vi "WhiteScreenTest_Startup.vi"() -> (0 "ErrorOut":errorcluster)   [LabVIEW 2018] (continued)
  w115 = "FPGA1" ("name (unnamed)")
  w161 = cluster{"QElmnt":T47, "Data":variant} {"QElmnt"=enum."Spvsr_InitQ", "Data"=variant} ("Cluster")
  # "Remove ATA_RF_Acquisition folder from path"
  # "Remove VI from path"
  # "Remove ATA_RF_Acquisition folder from path"
  # "Remove VI from path"
  # "Remove ATA_RF_Acquisition folder from path"
  # "Remove VI from path"
  # "Remove ATA_RF_Acquisition folder from path"
  # "Remove VI from path"
  # "Note that the Main Queue is made available to the HW Loop (and other loops) for things such as Error Handling as well as for allowing the HW Loop to drive information back up to the Main Loop for tasks such as refreshing panel controls  based on a change in HW State (\"Run\" to \"Pause\" or \"Waiting on Trigger\" to \"Triggered\")"
  # "The Hypervisor is optional and allows for data logging of user and other system events.  This can be expanded upon to be called from anywhere in the software depending on how detailed the event logging requirements of the application.\n\nThe data type defined for the queue allows for a string for event name, time, variant data type for longer descriptors or data and the stop condition but this can be expanded to allow for any number of variables to be written.\n\nWith each call to Add, an event is added to the Queue that needs to be read off and written.  The HypervisorWrite.vi is called in a parallel loop below to log these events as they are added to the queue."
  # "Copyright © 2017 Epimedia, Inc. All Rights Reserved.\n\nThe Epimedia Application Library is Copyright © 2009-2017 Epimedia, Inc. \nAll Rights Reserved. Used under license."
  # "Cluster data flow is predominantly top to bottom with data being passed using queues.  The Event Structure drives the Main (Consumer) Loop which acts as the Supervisor or dominant loop in this architecture.  In doing so, it handles the functionality of the other loops in your program.  The Consumer Loop processes the 'event' and then if necessary, sends the Master Cluster or a sub-cluster by means of a queue down to the Hardware Loop.  The Hardware loop checks the queued event's data for new information and if there is none, uses the previous iteration's cluster from the Shift Register.  Depending on the mode/event of the Hardware loop, the Hardware Loop may need to update the Master Cluster and does so by pushing the Refresh Panel Queue event which passes the cluster up to the Consumer loop for processing and panel update.  Note that there is a Functional Global inside of the UpdateMasterCluster.vi that is used to maintain a copy of the Master Cluster in memory that can be accessed from anywhere in the software (subVIs included).  This is not always and is often quite unnecessary, but is shown to illustrate a way of passing data between loops without using a Queue.  This use of a FG is quite effective, but must be used with care in that you need to be cautious with where and how often you update the FG; too many writers can cause unpredictable and very challenging code to debug.  The Functional Global exists to allow for any point anywhere in the program and in any loop to grab a copy of your cluster.  This architecture is intended to be a solid starting point for most applications, but you will need to configure and tailor the framework for your specific application and the use of some of the concepts shown herein cannot and should not always be used precisely as shown or at all.\n\nGeneral Rules:\n\n- Don't touch your Hardware anywhere except the HW loop.\n- Try to dedicate loops to very specific tasks to compartmentalize your code as much as possible as this helps with readability and scalability.\n- Any and all periodic updates (logging to disk, graph updates to name two) should occur only in the GUI loop.  Periodic updates of front panel indicators in any other loop will cause unnecessary loop cycles.\n- State changes for the program (ie. Idle, Run, Stop, Error) are handled in the Main Loop only and the panel is updated accordingly. \n- Use the Refresh Panel case in the Main Loop to handle all state changes and Panel GUI configuration tasks (enable/disable controls, visible, colors, alarming, status indicators, etc.).\n- Most loops only run when called by event/queue at the prescribed rate of the software.  Depending on your application, timed or free-wheeling loops could be implemented here if desired, but free-wheeling loops can be inefficient if not carefully implemented.\n- There are a couple of cases such as InitSW that are currently only called upon initialization and never again as shown below and one could argue that they could be outside of the architecture, but if they are called once, they may need to be again, so it is helpful to include them in the overall architecture for potential future use.  An example of this would be InitHW as in the event of a HW failure resulting from poor configuration choices, it would be helpful to be able to call the InitHW case again to reinitialize the HW with new settings."
  n1 = Current VI's Path() -> (path=w75:path)
  n2 = Current VI's Path() -> (path=w81:path)
  n3 = Strip Path(path=w75) -> (stripped path=w74:path)  [unwired: 1 out]
  n4 = Strip Path(path=w81) -> (stripped path=w80:path)  [unwired: 1 out]
  n5 = Strip Path(path=w74) -> (stripped path=w73:path)  [unwired: 1 out]
  n6 = Current VI's Path() -> (path=w91:path)
  n7 = Current VI's Path() -> (path=w83:path)
  n8 = Strip Path(path=w80) -> (stripped path=w79:path)  [unwired: 1 out]
  n9 = Strip Path(path=w91) -> (stripped path=w90:path)  [unwired: 1 out]
  n10 = Strip Path(path=w83) -> (stripped path=w84:path)  [unwired: 1 out]
  n11 = flat-sequence {
    tunnel: [w166] -> w111
    tunnel: errorcluster {"status"=FALSE, "code"=0, "source"=""} ("ErrorIn") -> [w165]
    frame #0 {
      n12 = shared-variable ".\\Connex_Variables.lvlib\\10Hz_File_Refs"(T48 {"72Co_dset"=0, "84Co_dset"=0, "FileRef"=0} ("10Hz_File_Refs"), error in=w165) -> (error out=w166:errorcluster)
      n13 = local write "Exit"(FALSE ("Exit")) -> ()
    }
  }
  n14 = Strip Path(path=w90) -> (stripped path=w89:path)  [unwired: 1 out]
  n15 = Strip Path(path=w84) -> (stripped path=w85:path)  [unwired: 1 out]
  n16 = control-ref of="Power History 72 Co"() -> (w93:refnum<vi>)
  n17 = control-ref of="Power History 72 X"() -> (w94:refnum<vi>)
  n18 = control-ref of="Power History 84 Co"() -> (w95:refnum<vi>)
  n19 = control-ref of="Power History 84 X"() -> (w96:refnum<vi>)
  n20 = Build Path(base path=w79, name or relative path="NASA\\wtle_young_weather_stn\\WeatherStationMain_20180517.vi") -> (appended path=w77:path)
  n21 = Build Path(base path=w73, name or relative path="NASA\\statmon_2015\\ADAM_health_subpanel_20190329.vi") -> (appended path=w71:path)
  n22 = Obtain Queue(max queue size (-1, unlimited)=100, name (unnamed)="Supervisor", element data type=w161, error in (no error)=w111) -> (queue out=w162:refnum<queue>, error out=w163:errorcluster)  [unwired: 1 in, 1 out]
  n23 = Build Array(w93, w94, w95, w96) -> (w92:refnum<vi>[])
  n24 = Build Path(base path=w89, name or relative path="Disdrometer\\disdrometer_2020_09_09.vi") -> (appended path=w87:path)
  n25 = Build Path(base path=w85, name or relative path="NASA\\te_2015\\te_20200903.vi") -> (appended path=w82:path)
  n26 = Enqueue Element(queue=w162, element=w161, error in (no error)=w163) -> (queue out=w144:refnum<queue>, error out=w57:errorcluster)  [unwired: 2 out]
  n27 = Open VI Reference(vi path=w71, error in (no error)=w57) -> (vi reference=w63:refnum<vi>, error out=w30:errorcluster)  [unwired: 4 in]
  n28 = Open VI Reference(vi path=w87, error in (no error)=w57) -> (vi reference=w62:refnum<vi>, error out=w45:errorcluster)  [unwired: 4 in]
  n29 = Open VI Reference(vi path=w82, error in (no error)=w57) -> (vi reference=w61:refnum<vi>, error out=w28:errorcluster)  [unwired: 4 in]
  n30 = Open VI Reference(vi path=w77, error in (no error)=w57) -> (vi reference=w4:refnum<vi>, error out=w16:errorcluster)  [unwired: 4 in]
  n31 = invoke on="DisdroPanel" class="SubPnl" method="Insert VI"(error in=w45, "VI Ref"=w62) -> (error out=w42:errorcluster)  [unwired: 2 in, 3 out]
  n32 = invoke on="TE_panel" class="SubPnl" method="Insert VI"(error in=w28, "VI Ref"=w61) -> (error out=w18:errorcluster)  [unwired: 2 in, 3 out]
  n33 = invoke on="Sub Panel - Weather" class="SubPnl" method="Insert VI"(error in=w16, "VI Ref"=w4) -> (error out=w6:errorcluster)  [unwired: 2 in, 3 out]
  n34 = Obtain Queue(max queue size (-1, unlimited)=100, name (unnamed)="Data", element data type=w118, error in (no error)=w57) -> (queue out=w122:refnum<queue>, error out=w120:errorcluster)  [unwired: 1 in, 1 out]
  n35 = Obtain Queue(max queue size (-1, unlimited)=110, name (unnamed)="FP", element data type=w97, error in (no error)=w57) -> (queue out=w100:refnum<queue>, error out=w99:errorcluster)  [unwired: 1 in, 1 out]
  n36 = invoke on="ADAM Health" class="SubPnl" method="Insert VI"(error in=w30, "VI Ref"=w63) -> (error out=w29:errorcluster)  [unwired: 2 in, 3 out]
  n37 = Obtain Queue(max queue size (-1, unlimited)=100, name (unnamed)=w115, element data type=cluster{"HWMd":T27, "Data":variant} {"HWMd"=enum."HW_Init", "Data"=variant}, error in (no error)=w57) -> (queue out=w150:refnum<queue>, error out=w149:errorcluster)  [unwired: 1 in, 1 out]
  n38 = Obtain Queue(max queue size (-1, unlimited)=100, name (unnamed)=w114, element data type=cluster{"HWMd":T27, "Data":variant} {"HWMd"=enum."HW_Init", "Data"=variant}, error in (no error)=w57) -> (queue out=w53:refnum<queue>, error out=w131:errorcluster)  [unwired: 1 in, 1 out]
  n39 = Enqueue Element(queue=w122, element=w118, error in (no error)=w120) -> (queue out=w121:refnum<queue>, error out=w119:errorcluster)  [unwired: 1 in, 1 out]
  n40 = Obtain Queue(max queue size (-1, unlimited)=100, name (unnamed)="10Hz", element data type=cluster{"Enum":T23, "Var":variant} {"Enum"=enum."10Hz_Init", "Var"=variant}) -> (queue out=w2:refnum<queue>, error out=w3:errorcluster)  [unwired: 2 in, 1 out]
  n41 = Obtain Queue(max queue size (-1, unlimited)=1000, name (unnamed)="Tones", element data type=cluster{"Enum":T46, "Data":variant} {"Enum"=enum."Data_Init", "Data"=variant}, error in (no error)=w57) -> (queue out=w145:refnum<queue>, error out=w156:errorcluster)  [unwired: 1 in, 1 out]
  n42 = Obtain Queue(max queue size (-1, unlimited)=100, name (unnamed)="Digi", element data type=w124, error in (no error)=w57) -> (queue out=w128:refnum<queue>, error out=w126:errorcluster)  [unwired: 1 in, 1 out]
  n43 = Obtain Queue(max queue size (-1, unlimited)=100, name (unnamed)="Log", element data type=w65, error in (no error)=w57) -> (queue out=w67:refnum<queue>, error out=w69:errorcluster)  [unwired: 1 in, 1 out]
  n44 = Enqueue Element(queue=w100, element=w97, error in (no error)=w99) -> (queue out=w70:refnum<queue>, error out=w98:errorcluster)  [unwired: 1 in, 1 out]
  n45 = Enqueue Element(queue=w67, element=w65, error in (no error)=w69) -> (queue out=w66:refnum<queue>, error out=w68:errorcluster)  [unwired: 1 in, 1 out]
  n46 = invoke class="VI" method="Run VI"(reference=w4, error in=w6, "Wait until done"=FALSE ("Wait Until Done"), "Auto Dispose Ref"=FALSE ("Auto Dispose Reference")) -> (error out=w5:errorcluster)  [unwired: 1 in, 4 out]
  n47 = invoke class="VI" method="Run VI"(reference=w63, error in=w29, "Wait until done"=FALSE ("Wait Until Done"), "Auto Dispose Ref"=FALSE ("Auto Dispose Reference")) -> (error out=w31:errorcluster)  [unwired: 1 in, 4 out]
  n48 = invoke class="VI" method="Run VI"(reference=w62, error in=w42, "Wait until done"=FALSE ("Wait Until Done"), "Auto Dispose Ref"=FALSE ("Auto Dispose Reference")) -> (error out=w41:errorcluster)  [unwired: 1 in, 4 out]
  n49 = invoke class="VI" method="Run VI"(reference=w61, error in=w18, "Wait until done"=FALSE ("Wait Until Done"), "Auto Dispose Ref"=FALSE ("Auto Dispose Reference")) -> (error out=w17:errorcluster)  [unwired: 1 in, 4 out]
  n50 = Enqueue Element(queue=w128, element=w124, error in (no error)=w126) -> (queue out=w127:refnum<queue>, error out=w125:errorcluster)  [unwired: 1 in, 1 out]
  n51 = call "NoiseLoop.vi"("error in (no error)"=w119, "Queue in"=w121) -> ("error out"=w143:errorcluster)  [unwired: 9 in]
  n52 = disable-structure shown="Enabled" {
    disable-tunnel: [w173 w174] -> w117
    disable-tunnel: [w170 w174] -> w110
    disable-tunnel: w57 -> [w169 w174]
    frame Enabled {
      n53 = call "AI_Loop.vi"("error in"=w169, "AI_Type"=AI_Type_Enum."AI") -> ("error out"=w173:errorcluster)  [unwired: 9 in]
      n54 = call "AI_Loop.vi"("error in"=w169, "AI_Type"=AI_Type_Enum."TC") -> ("error out"=w170:errorcluster)  [unwired: 9 in]
    }
    frame Disabled {
    }
  }
  n55 = disable-structure shown="Enabled" {
    disable-tunnel: [w176 w177] -> w108
    disable-tunnel: w57 -> [w175 w177]
    frame Enabled {
      n56 = call "AO_Loop.vi"("error"=w175) -> ("error out"=w176:errorcluster)  [unwired: 10 in]
    }
    frame Disabled {
    }
  }
  n57 = call "LogLoop_HDF5_20190307.vi"("error in"=w68, "Queue in"=w66) -> ("error out"=w107:errorcluster)  [unwired: 9 in]
  n58 = call "DigitalOutput.vi"("error in (no error)"=w125, "Queue in"=w127) -> ("error out"=w116:errorcluster)  [unwired: 9 in]
  n59 = call "10HzLogLoop_HDF5_20210610.vi"("error in"=w3, "queue in"=w2) -> ("error out"=w54:errorcluster)  [unwired: 9 in]
  n60 = while {
    tunnel: w57 -> [w180]
    tunnel: [w178] -> w104
    stop <- w183 stop-if-true
    n61 = call "Elapsed Time"("Time Target (s)"="MemoryPlotRate") -> ("Time has Elapsed"=w182:bool)  [unwired: 11 in, 7 out]
    n62 = Wait Until Next ms Multiple(millisecond multiple=u32 50) -> ()  [unwired: 1 out]
    n63 = case shown="True" w182 {
      tunnel: w180 -> [w184 w187]
      tunnel: [w184 w185] -> w178
      frame False {
      }
      frame True {
        n64 = constructor class="Process"(error in=w187) -> (reference out=w197:refnum<k24>, error out=w188:errorcluster)  [unwired: 2 in, 1 out]
        n65 = invoke class="Process" method="GetCurrentProcess"(reference=w197, error in=w188) -> (reference out=w195:refnum<k24>, error out=w196:errorcluster, "GetCurrentProcess"=w189:refnum<k24>)  [unwired: 1 in]
        n66 = property class="Process"(reference=w189, error in=w196) -> (reference out=w193:refnum<k24>, error out=w192:errorcluster, "WorkingSet"=w190:i32)
        n67 = Divide(x=w190, y=i64 1024) -> (x/y=→"Memory Used By LV (KB)" →"Memory Used":dbl)
        n68 = Close Reference(reference=w193, error in (no error)=w192) -> (error out=w194:errorcluster)
        n69 = Close Reference(reference=w195, error in (no error)=w194) -> (error out=w185:errorcluster)
      }
    }
    n70 = local read "Exit"() -> (w183:bool)
  }
  n71 = call "TonesLoop_20190705.vi"("WeightOfNewFrequency"=1.0, "error in"=w156, "Queue in"=w145) -> ("error out"=w146:errorcluster)  [unwired: 8 in]
  n72 = while {
    tunnel: w144 -> [w201]
    shift-right: [w200] -> w155
    shift-left: w57 -> [w202]
    stop <- w199 stop-if-true
    n73 = event shown="[14] \"Exit\": Value Change;  Panel Close" {
      selector: _ -> [_ _ _ _ _ _ _ _ _ _ _ _ _ _ _]
      dyn-events: _ -> [_ _ _ _ _ _ _ _ _ _ _ _ _ _ _]
      timeout: 100 -> [_ _ _ _ _ _ _ _ _ _ _ _ _ _ _]
      tunnel: w202 -> [w207 w211 w220 w228 w234 w236 w240 w248 w256 w264 w267 w272 w276 w280 w284]
      tunnel: w201 -> [_ w218 w221 w223 w229 w237 w241 w249 w257 w265 w269 w273 w277 w281 w286]
      tunnel: [w207 w210 w222 w224 w230 w235 w239 w247 w255 w263 w268 w271 w275 w282 w285] -> w200
      tunnel: [_ w209 _ _ _ _ _ _ _ _ _ _ _ _ TRUE] -> w199
      event Timeout {
        # "13:24:24.3\n05/31/2018"
        # "Timeout Case is used to update 'heartbeat' clock on the front panel to provide an indication that the software is still running"
        n74 = event-data() -> ()  [unwired: 2 out]
        n75 = Get Date/Time In Seconds() -> (seconds since 1Jan1904=w206:timestamp)
        n76 = Format Date/Time String(time format string (%c)="%H:%M:%S%1u\n%m/%d/%Y", seconds (now)=w206, UTC format=TRUE) -> (date/time string=→"UTC date/time":string)
      }
      event Menu Selection (User) {
        # "This handles a menu selection while the program is running."
        n77 = event-data() -> ("ItemTag"=w212:string)  [unwired: 1 out]
        n78 = Scan From String(input string=w212, error in=w211, default 1=MainQueueElements."Spvsr_InitQ" ("QElmnt")) -> (error out=w208:errorcluster, output 1=w216:T47)  [unwired: 2 in, 2 out]
        n79 = Bundle(cluster=cluster{"QElmnt":T47, "Data":variant} {"QElmnt"=enum."Spvsr_InitQ", "Data"=variant} ("Cluster"), "QElmnt"=w216) -> (w215:cluster{"QElmnt":T47, "Data":variant})  [unwired: 1 in]
        n80 = Enqueue Element(queue=w218, element=w215, error in (no error)=w208) -> (error out=w210:errorcluster)  [unwired: 3 out]
        n81 = Equal?(x=MainQueueElements."Spvsr_Exit" ("QElmnt"), y=w216) -> (x = y?=w209:bool)
      }
      event Value Change {
        n82 = event-data() -> ()  [unwired: 2 out]
        n83 = Enqueue Element(queue=w221, element=cluster{"QElmnt":T51, "Data":variant} {"QElmnt"=enum."Spvsr_DigiOut", "Data"=variant} ("Cluster"), error in (no error)=w220) -> (error out=w222:errorcluster)  [unwired: 3 out]
      }
      event "Config": Value Change {
        n84 = event-data() -> ()  [unwired: 2 out]
        n85 = Enqueue Element(queue=w223, element=cluster{"QElmnt":T47, "Data":variant} {"QElmnt"=enum."Spvsr_Config", "Data"=variant} ("Cluster"), error in (no error)=w228) -> (error out=w225:errorcluster)  [unwired: 3 out]
        n86 = Enqueue Element(queue=w223, element=cluster{"QElmnt":T47, "Data":variant} {"QElmnt"=enum."Spvsr_FPConfig", "Data"=variant} ("Cluster"), error in (no error)=w225) -> (error out=w224:errorcluster)  [unwired: 3 out]
      }
      event "AutoOffset": Value Change {
        n87 = event-data() -> ()  [unwired: 2 out]
        n88 = Enqueue Element(queue=w229, element=cluster{"QElmnt":T47, "Data":variant} {"QElmnt"=enum."Spvsr_DigitzOffs", "Data"=variant} ("Cluster"), error in (no error)=w234) -> (error out=w231:errorcluster)  [unwired: 3 out]
        n89 = Enqueue Element(queue=w229, element=cluster{"QElmnt":T47, "Data":variant} {"QElmnt"=enum."Spvsr_FPConfig", "Data"=variant} ("Cluster"), error in (no error)=w231) -> (error out=w230:errorcluster)  [unwired: 3 out]
      }
      event "FreqsToRemove", "AvgAvg", "SNR_Thresh", "Width [bins]", "FreqsToRemove 2", "Width 2 [bins]", "SimulateFPGA": Value Change {
        n90 = event-data() -> ()  [unwired: 2 out]
        n91 = Enqueue Element(queue=w237, element=cluster{"QElmnt":T47, "Data":variant} {"QElmnt"=enum."Spvsr_FPConfig", "Data"=variant} ("Cluster"), error in (no error)=w236) -> (error out=w235:errorcluster)  [unwired: 3 out]
      }
      event "MaxTrackRate": Value Change {
        n92 = event-data() -> ()  [unwired: 6 out]
        n93 = for {
          tunnel: cluster{"QElmnt":T47, "Data":variant}[] [{"QElmnt"=enum."Spvsr_FPConfig", "Data"=variant}, {"QElmnt"=enum."Spvsr_TrackRate", "Data"=variant}] ("Cluster") -> [w245] mode=indexing
          tunnel: w241 -> [w244]
          shift-right: [w243] -> w239
          shift-left: w240 -> [w246]
          n94 = Enqueue Element(queue=w244, element=w245, error in (no error)=w246) -> (error out=w243:errorcluster)  [unwired: 3 out]
        }
      }
      event "AutoCenter": Value Change {
        n95 = event-data() -> ()  [unwired: 6 out]
        n96 = for {
          tunnel: cluster{"QElmnt":T47, "Data":variant}[] [{"QElmnt"=enum."Spvsr_FPConfig", "Data"=variant}, {"QElmnt"=enum."Spvsr_AutoCenter", "Data"=variant}] ("Cluster") -> [w253] mode=indexing
          tunnel: w249 -> [w252]
          shift-right: [w251] -> w247
          shift-left: w248 -> [w254]
          n97 = Enqueue Element(queue=w252, element=w253, error in (no error)=w254) -> (error out=w251:errorcluster)  [unwired: 3 out]
        }
      }
      event "base path", "NAS path", "ThreshFile", "Location": Value Change {
        n98 = event-data() -> ()  [unwired: 6 out]
        n99 = for {
          tunnel: cluster{"QElmnt":T47, "Data":variant}[] [{"QElmnt"=enum."Spvsr_FPConfig", "Data"=variant}, {"QElmnt"=enum."Spvsr_RestartWarn", "Data"=variant}] ("Cluster") -> [w261] mode=indexing
          tunnel: w257 -> [w260]
          shift-right: [w259] -> w255
          shift-left: w256 -> [w262]
          n100 = Enqueue Element(queue=w260, element=w261, error in (no error)=w262) -> (error out=w259:errorcluster)  [unwired: 3 out]
        }
      }
      event "Beacon", "Beacon 3": Cursor Move {
        n101 = event-data() -> ()  [unwired: 2 out]
        n102 = Enqueue Element(queue=w265, element=cluster{"QElmnt":T47, "Data":variant} {"QElmnt"=enum."Spvsr_Cursors", "Data"=variant} ("Cluster"), error in (no error)=w264) -> (error out=w263:errorcluster)  [unwired: 3 out]
      }
      event "noise_ctrl", "72GHz_ctrl", "84GHz_ctrl": Value Change {
        n103 = event-data() -> ()  [unwired: 6 out]
        n104 = Enqueue Element(queue=w269, element=cluster{"QElmnt":T47, "Data":variant} {"QElmnt"=enum."FP_AO_ctrl", "Data"=variant} ("Cluster"), error in (no error)=w267) -> (error out=w268:errorcluster)  [unwired: 3 out]
      }
      event "Zoom On Peak", "AutoScale Y Noise", "AutoScale Y Tones": Value Change {
        n105 = event-data() -> ()  [unwired: 2 out]
        n106 = Enqueue Element(queue=w273, element=cluster{"QElmnt":T47, "Data":variant} {"QElmnt"=enum."Spvsr_FPConfig", "Data"=variant} ("Cluster"), error in (no error)=w272) -> (error out=w271:errorcluster)  [unwired: 3 out]
      }
      event Value Change {
        n107 = event-data() -> ()  [unwired: 6 out]
        n108 = Enqueue Element(queue=w277, element=cluster{"QElmnt":T47, "Data":variant} {"QElmnt"=enum."Spvsr_AlarmCfg", "Data"=variant} ("Cluster"), error in (no error)=w276) -> (error out=w275:errorcluster)  [unwired: 3 out]
      }
      event "Stop": Value Change {
        n109 = event-data() -> ()  [unwired: 2 out]
        n110 = Enqueue Element(queue=w281, element=cluster{"QElmnt":T47, "Data":variant} {"QElmnt"=enum."Spvsr_Stop", "Data"=variant} ("Cluster"), error in (no error)=w280) -> (error out=w282:errorcluster)  [unwired: 3 out]
      }
      event "Exit": Value Change; Panel Close {
        n111 = event-data() -> ()  [unwired: 2 out]
        n112 = Enqueue Element(queue=w286, element=cluster{"QElmnt":T47, "Data":variant} {"QElmnt"=enum."Spvsr_Exit", "Data"=variant} ("Cluster"), error in (no error)=w284) -> (error out=w285:errorcluster)  [unwired: 3 out]
      }
    }
  }
  n113 = while {
    shift-right: [w301] -> w154
    shift-left: w57 -> [w300]
    tunnel: w144 -> [w291]
    shift-right: [w302] -> _
    shift-left: T32 {"Admin"={"Lvl"=enum."Admin", "Pwd"=""}, "RTConfig"={"Arm"=FALSE, "Number"=0.0, "String"=""}, "SMS"={"Enbl?"=FALSE, "Addr"=[]}, "FPGA"={"Target"=enum."1", "Channel"=enum."1", "Ref1"=refnum, "Ref2"=refnum}, "Config"={"UsrCfg"={"Paths"={"CfgFile"=path "", "LogFolder"=path "", "LogFile"=path "", "NAS path"=path "", "ThreshFile"=path "", "RedunFolder"=path ""}, "SampleRate"=0.0}, "FP_User"={"#NoiseSums"=0, "Max_df"=0, "AvgAvg"=FALSE, "#Avg"=0, "AutoCenter"=FALSE, "Inclin"={"Vmin"=0.0, "Vmax"=0.0, "Angle_min"=0.0, "Angle_max"=0.0, "Offset"=0.0, "Pos_Neg"=FALSE}, "1"={"Cal_"={"Fine"=0.0, "Coarse_"=0.0}, "Beac"={"Fine"=0.0, "Coarse_"=0.0}, "Scale"={"Step4"=0.0, "Step5"=0.0, "Step6"=0.0, "Step7"=0.0}, "Offset"=0.0, "Scale_Noise"=0.0, "Scale_Step1"=0.0, "Scale_In_RT"=0.0, "ScaleMeas"=0.0, "FreqsToRemove"=[], "Width"=[], "ScaleMeasEnum"=enum."1", "FilterEnab"=enum."None"}, "2"={"Cal_"={"Fine"=0.0, "Coarse_"=0.0}, "Beac"={"Fine"=0.0, "Coarse_"=0.0}, "Scale"={"Step4"=0.0, "Step5"=0.0, "Step6"=0.0, "Step7"=0.0}, "Offset"=0.0, "Scale_Noise"=0.0, "Scale_Step1"=0.0, "Scale_In_RT"=0.0, "ScaleMeas"=0.0, "FreqsToRemove"=[], "Width"=[], "ScaleMeasEnum"=enum."1", "FilterEnab"=enum."None"}, "3"={"Cal_"={"Fine"=0.0, "Coarse_"=0.0}, "Beac"={"Fine"=0.0, "Coarse_"=0.0}, "Scale"={"Step4"=0.0, "Step5"=0.0, "Step6"=0.0, "Step7"=0.0}, "Offset"=0.0, "Scale_Noise"=0.0, "Scale_Step1"=0.0, "Scale_In_RT"=0.0, "ScaleMeas"=0.0, "FreqsToRemove"=[], "Width"=[], "ScaleMeasEnum"=enum."1", "FilterEnab"=enum."None"}, "4"={"Cal_"={"Fine"=0.0, "Coarse_"=0.0}, "Beac"={"Fine"=0.0, "Coarse_"=0.0}, "Scale"={"Step4"=0.0, "Step5"=0.0, "Step6"=0.0, "Step7"=0.0}, "Offset"=0.0, "Scale_Noise"=0.0, "Scale_Step1"=0.0, "Scale_In_RT"=0.0, "ScaleMeas"=0.0, "FreqsToRemove"=[], "Width"=[], "ScaleMeasEnum"=enum."1", "FilterEnab"=enum."None"}, "Target to Probe"=enum."1", "SNR_Thresh"=0.0, "Paths"={"CfgFile"=path "", "LogFolder"=path "", "LogFile"=path "", "NAS path"=path "", "ThreshFile"=path "", "RedunFolder"=path ""}, "Connex_Location"="", "SimulateFPGA"=FALSE}}, "Stat"={"SysState"=enum."Init", "TrackRate"=FALSE, "AutoCentr"=FALSE}, "Alarm"={"TC13"={"Enbl"=FALSE, "ErrsAndWarns"={0.0, 0.0, 0.0, 0.0}}, "AI1"={"Enbl"=FALSE, "ErrsAndWarns"={0.0, 0.0, 0.0, 0.0}}, "AI2"={"Enbl"=FALSE, "ErrsAndWarns"={0.0, 0.0, 0.0, 0.0}}, "AI3"={"Enbl"=FALSE, "ErrsAndWarns"={0.0, 0.0, 0.0, 0.0}}, "AI4"={"Enbl"=FALSE, "ErrsAndWarns"={0.0, 0.0, 0.0, 0.0}}, "AI5"={"Enbl"=FALSE, "ErrsAndWarns"={0.0, 0.0, 0.0, 0.0}}, "AI6"={"Enbl"=FALSE, "ErrsAndWarns"={0.0, 0.0, 0.0, 0.0}}, "AI18"={"Enbl"=FALSE, "ErrsAndWarns"={0.0, 0.0, 0.0, 0.0}}, "AI19"={"Enbl"=FALSE, "ErrsAndWarns"={0.0, 0.0, 0.0, 0.0}}, "TE1"={"Enbl"=FALSE, "ErrsAndWarns"={0.0, 0.0, 0.0, 0.0}}, "TE2"={"Enbl"=FALSE, "ErrsAndWarns"={0.0, 0.0, 0.0, 0.0}}, "TE3"={"Enbl"=FALSE, "ErrsAndWarns"={0.0, 0.0, 0.0, 0.0}}, "ADAM1"={"Enbl"=FALSE, "ErrsAndWarns"={0.0, 0.0, 0.0, 0.0}}, "ADAM2"={"Enbl"=FALSE, "ErrsAndWarns"={0.0, 0.0, 0.0, 0.0}}, "ADAM3"={"Enbl"=FALSE, "ErrsAndWarns"={0.0, 0.0, 0.0, 0.0}}, "ADAM4"={"Enbl"=FALSE, "ErrsAndWarns"={0.0, 0.0, 0.0, 0.0}}, "72CoBeacFreq"={"Enbl"=FALSE, "ErrsAndWarns"={0.0, 0.0, 0.0, 0.0}}, "72CoCalFreq"={"Enbl"=FALSE, "ErrsAndWarns"={0.0, 0.0, 0.0, 0.0}}, "84CoBeacFreq"={"Enbl"=FALSE, "ErrsAndWarns"={0.0, 0.0, 0.0, 0.0}}, "84CoCalFreq"={"Enbl"=FALSE, "ErrsAndWarns"={0.0, 0.0, 0.0, 0.0}}, "72Co_CalTonePwr"={"Enbl"=FALSE, "ErrsAndWarns"={0.0, 0.0, 0.0, 0.0}}, "72X_CalTonePwr"={"Enbl"=FALSE, "ErrsAndWarns"={0.0, 0.0, 0.0, 0.0}}, "84Co_CalTonePwr"={"Enbl"=FALSE, "ErrsAndWarns"={0.0, 0.0, 0.0, 0.0}}, "84X_CalTonePwr"={"Enbl"=FALSE, "ErrsAndWarns"={0.0, 0.0, 0.0, 0.0}}}} ("ClusterIn") -> [w309]
    tunnel: w150 -> [w297]
    tunnel: w145 -> [w296]
    tunnel: w121 -> [w295]
    tunnel: w66 -> [w294]
    tunnel: w70 -> [w293]
    tunnel: w2 -> [w289]
    tunnel: w53 -> [w288]
    i -> [w292]
    stop <- w308 stop-if-true
    # "MasterCluster"
    # "Main \n(Supervisor)\nLoop"
    # "Supervisor Loop"
    n114 = call "PushToErrorHandler.vi"("ErrorIn"=w300, "ErrorLocation"="Supervisor") -> ("ErrorOut"=w299:errorcluster)  [unwired: 5 in]
    n115 = Get Queue Status(queue=w291) -> (# elements in queue=→"SPVSR_Queue":i32)  [unwired: 2 in, 7 out]
    n116 = Dequeue Element(queue=w291, error in (no error)=w299) -> (queue out=w307:refnum<queue>, element=w305:cluster{"QElmnt":T47, "Data":variant}, error out=w306:errorcluster)  [unwired: 2 out]
    n117 = Unbundle(w305) -> ("QElmnt"=w304:T47, "Data"=w303:variant)
    n118 = case shown="\"Spvsr_InitSW\"" w304 {
      tunnel: w306 -> [w320 w328 w407 w416 w450 w456 w484 w509 w516 w520 w530 w603 w666 w694 w713 w748 w775 w844 w848 w850 w869 w902 w904]
      tunnel: [w319 w353 w401 w415 w448 w462 w481 w511 w513 w521 w534 w598 w619 w696 w721 w739 w774 w843 w847 w851 w854 w900 w908] -> w302
      tunnel: w309 -> [w319 w354 w401 w418 w448 w463 w481 w512 w513 w521 w535 w604 w609 w693 w720 w739 w774 w842 w846 w851 w866 w900 w908]
      tunnel: [_ _ _ _ _ _ _ _ _ _ _ _ _ _ _ _ _ _ _ _ _ _ TRUE] -> w308
      tunnel: [w318 w355 w407 w412 w439 w457 w482 w506 w515 w520 w537 w600 w665 w690 w713 w734 w775 w844 w848 w850 w853 w901 w905] -> w301
      tunnel: w307 -> [w321 _ _ _ _ w453 _ w507 _ _ w531 _ _ _ _ _ _ _ _ _ w876 _ _]
      tunnel: w303 -> [_ _ _ w417 _ _ _ _ w514 _ w532 _ _ _ _ _ _ _ _ _ _ _ _]
      tunnel: w297 -> [_ _ _ _ _ _ _ _ _ _ w536 _ _ _ _ _ _ _ _ _ _ _ _]
      tunnel: w296 -> [_ _ _ _ _ _ _ _ _ _ _ _ w664 _ _ _ _ _ _ _ _ _ w907]
      tunnel: w295 -> [_ _ _ _ _ _ _ _ _ _ _ _ w659 _ _ _ _ _ _ _ _ _ w906]
      tunnel: w294 -> [_ _ _ _ _ _ _ _ _ _ _ _ w635 w689 _ w733 _ _ _ _ _ _ _]
      tunnel: w293 -> [_ _ _ _ _ _ _ _ _ _ _ _ _ _ _ _ _ _ _ _ _ _ _]
      tunnel: w289 -> [_ _ _ _ _ _ _ _ _ _ _ _ _ _ _ _ _ _ _ _ _ _ w903]
      tunnel: w288 -> [_ _ _ _ _ _ _ _ _ _ _ _ _ _ _ _ _ _ _ _ _ _ _]
      frame "Spvsr_InitQ" {
        # "This case is called upon launch and calls all cases necessary to initialize the application."
        n119 = Build Array(cluster{"QElmnt":T47, "Data":variant} {"QElmnt"=enum."Spvsr_InitSW", "Data"=variant} ("Cluster"), cluster{"QElmnt":T47, "Data":variant} {"QElmnt"=enum."Spvsr_InitCtrls", "Data"=variant} ("Cluster"), cluster{"QElmnt":T47, "Data":variant} {"QElmnt"=enum."Spvsr_FPConfig", "Data"=variant} ("Cluster"), cluster{"QElmnt":T47, "Data":variant} {"QElmnt"=enum."Spvsr_AlarmCfg", "Data"=variant} ("Cluster"), cluster{"QElmnt":T47, "Data":variant} {"QElmnt"=enum."Spvsr_StrtHWLp", "Data"=variant} ("Cluster"), cluster{"QElmnt":T47, "Data":variant} {"QElmnt"=enum."Spvsr_RfrshPnl", "Data"=variant} ("Cluster"), cluster{"QElmnt":T47, "Data":variant} {"QElmnt"=enum."Spvsr_ChkTime", "Data"=variant} ("Cluster")) -> (w312:cluster{"QElmnt":T47, "Data":variant}[])
        n120 = for {
          tunnel: w321 -> [w325]
          tunnel: w312 -> [w322] mode=indexing
          shift-right: [w323] -> w318
          shift-left: w320 -> [w324]
          n121 = Enqueue Element(queue=w325, element=w322, error in (no error)=w324) -> (error out=w323:errorcluster)  [unwired: 1 in, 2 out]
        }
      }
      frame "Spvsr_InitSW" {
        # "These files are updated in the tones (Data) loop"
        # "This case is used to initialize the startup conditions for your software."
        n122 = call "MountNAS.vi"("error in"=w328) -> ("error out"=w327:errorcluster)  [unwired: 10 in]
        n123 = call "InitSupervisorCluster.vi"("error in (no error)"=w327, "ClusterIn in"=w354) -> ("error out"=w331:errorcluster, "ClusterIn out"=w358:T32)  [unwired: 8 in]
        n124 = call "PushToErrorHandler.vi"("ErrorIn"=w331, "ErrorLocation"="InitClust") -> ("ErrorOut"=w330:errorcluster)  [unwired: 5 in]
        n125 = call "ReadConfigFile.vi"("ErrorIn"=w330, "ClusterIn"=w358) -> ("ErrorOut"=w335:errorcluster, "dup path"=w338:path, "ClusterOut"=w337:T32)  [unwired: 1 in, 6 out]
        n126 = call "ReadThreshFile_20200519.vi"("MainClust"=w337) -> ("ErrorOut"=w334:errorcluster, "dup path"=w333:path, "MainClustOut"=w336:T32)  [unwired: 8 in]
        n127 = case shown="Error" w335 {
          tunnel: w338 -> [_ w370]
          frame No Error {
          }
          frame Error {
            # "This triggers the\n\"exit\" event."
            n128 = property on="Exit" class="Bool (strict)"("Val(Sgnl)"=TRUE ("Value (Signaling)")) -> ()  [unwired: 2 in, 2 out]
            n129 = Path To String(path=w370) -> (string=w369:string)
            n130 = Concatenate Strings("Unfortunately, there is a problem with your configuration file.\nThis software will not run properly with the configuration file you have. \n\nYou can likely fix the problem by simply renaming your existing file and reconfiguring the system. \n\nThe file is found at:", w369, "\r\n", "For help with this, please contact Epimedia at 1.888.374.6334\n\nError 1108 " ("string")) -> (w366:string)
            n131 = One Button Dialog(message=w366) -> ()  [unwired: 1 in, 1 out]
          }
        }
        n132 = case shown="Error" w334 {
          tunnel: w333 -> [_ w363]
          frame No Error {
          }
          frame Error {
            n133 = Path To String(path=w363) -> (string=w362:string)
            n134 = Concatenate Strings("Unfortunately, there is a problem with your thresholds file.\nThis software will not run properly with the thresholds file you have. \n\nThe file is expected at:", w362, "\r\n", "For help with this, please contact Epimedia at 1.888.374.6334\n\nError 1109 " ("string")) -> (w359:string)
            n135 = One Button Dialog(message=w359) -> ()  [unwired: 1 in, 1 out]
          }
        }
        n136 = call <vilib>:"Clear Errors.vi"("error in (no error)"=w334) -> ("error out"=w332:errorcluster)  [unwired: 5 in, 1 out]
        n137 = call "InitFreqFiles.vi"("error in"=w332, "FileName"="72.txt") -> ("error out"=w348:errorcluster, "value"=w339:dbl)  [unwired: 7 in, 1 out]
        n138 = Subtract(x=w339, y=2500.0 ("x")) -> (x-y=w340:dbl)
        n139 = call "InitFreqFiles.vi"("error in"=w348, "FileName"="84.txt") -> ("error out"=w326:errorcluster, "value"=w347:dbl)  [unwired: 7 in, 1 out]
        n140 = Bundle By Name(cluster=T11 {"Fine"=0.0, "Coarse_"=0.0} ("72 Beac"), "Coarse_"=w340) -> (w346:T11)
        n141 = Subtract(x=w347, y=2500.0 ("x")) -> (x-y=w343:dbl)
        n142 = Bundle By Name(cluster=T11 {"Fine"=0.0, "Coarse_"=0.0} ("72 Beac"), "Coarse_"=w343) -> (w345:T11)
        n143 = Bundle By Name(cluster=w336, "Config.FP_User.Max_df"=u32 1, "Config.FP_User.1.Beac"=w346, "Config.FP_User.2.Beac"=w346, "Config.FP_User.3.Beac"=w345, "Config.FP_User.4.Beac"=w345) -> (w353:T32)
        n144 = Not(x=TRUE ("Visible")) -> (.not. x?=w356:bool)
        n145 = property on="Stop" class="Bool"(error in=w326, "Visible"=w356) -> (error out=w355:errorcluster)  [unwired: 1 in, 1 out]
      }
      frame "Spvsr_InitCtrls" {
        w400 = TRUE ("72GHz_ctrl")
        # "Distinct \"Redundant Folder\" no longer used."
        # "# of sums of noise floor to be recorded is no longer user-configurable. Always 86,400"
        # "# Averages in FPGA no longer user configurable. Always 150."
        # "Cal shift is recorded as a negative value and must be corrected here for display.\nBeac shift is changed to positive before it is recorded."
        # "Auto Center must be off at startup. FFT is nonsense at startup. Auto Center will jump to 0 and never move."
        # "Initalize controls with values from config file."
        n146 = Unbundle By Name(w401) -> ("Config.FP_User.AvgAvg"=w406:bool, "Config.FP_User.1.Cal_"=w405:T11, "Config.FP_User.1.Beac"=w404:T11, "Config.FP_User.1.FilterEnab"=w388:T6, "Config.FP_User.1.ScaleMeas"=w397:fxp<+/-,16,1>, "Config.FP_User.1.Scale_Step1"=w396:fxp<+/-,17,17>, "Config.FP_User.1.Scale"=w395:T5, "Config.FP_User.1.Offset"=w376:fxp<+/-,16,16>, "Config.FP_User.2.Offset"=w375:fxp<+/-,16,16>, "Config.FP_User.3.Offset"=w374:fxp<+/-,16,16>, "Config.FP_User.4.Offset"=w373:fxp<+/-,16,16>, "Config.FP_User.1.FreqsToRemove"=w403:i32[], "Config.FP_User.Target to Probe"=w402:T21, "Config.FP_User.3.FreqsToRemove"=w379:i32[], "Config.FP_User.3.Width"=w378:i32[], "Config.FP_User.SNR_Thresh"=w380:dbl, "Config.FP_User.Paths.LogFolder"=w389:path, "Config.FP_User.Paths.NAS path"=w390:path, "Config.FP_User.Paths.ThreshFile"=w391:path, "Config.FP_User.Connex_Location"=w392:string, "Config.FP_User.Max_df"=w393:u32, "Config.FP_User.1.Width"=w387:i32[], "Config.FP_User.Inclin"=w384:T8, "Alarm"=w381:T18)  [unwired: 5 out]
        n147 = local write "FilterEnable"(w388) -> ()
        n148 = local write "AvgAvg"(w406) -> ()
        n149 = local write "AutoCenter"(FALSE ("AutoCenter")) -> ()
        n150 = local write "AlarmSettings"(w381) -> ()
        n151 = local write "Width [bins]"(w387) -> ()
        n152 = Bundle By Name(cluster=T4 {"Measure"=0.050018310546875, "Step1"=2.0, "Scale"={"Step4"=3.0, "Step5"=1.0, "Step6"=1.0, "Step7"=1.0}} ("Scale"), "Measure"=w397, "Step1"=w396, "Scale"=w395) -> (w394:T4)
        n153 = local write "FreqsToRemove 2"(w379) -> ()
        n154 = local write "FreqsToRemove"(w403) -> ()
        n155 = local write "Target to Probe"(w402) -> ()
        n156 = local write "Width 2 [bins]"(w378) -> ()
        n157 = local write "SNR_Thresh"(w380) -> ()
        n158 = local write "base path"(w389) -> ()
        n159 = local write "NAS path"(w390) -> ()
        n160 = local write "ThreshFile"(w391) -> ()
        n161 = local write "Location"(w392) -> ()
        n162 = local write "MaxTrackRate"(w393) -> ()
        n163 = local write "Inclin"(w384) -> ()
        n164 = local write "Scale"(w394) -> ()
        n165 = local write "Digitizer Offset 72 Co"(w376) -> ()
        n166 = local write "Digitizer Offset 72 X"(w375) -> ()
        n167 = local write "Digitizer Offset 84 Co"(w374) -> ()
        n168 = local write "Digitizer Offset 84 x"(w373) -> ()
        n169 = Negate(x=w405) -> (-x=w383:T11)
        n170 = local write "RightSideTab"(T2."PXI" ("RightSideTab")) -> ()
        n171 = local write "Shift Cal"(w383) -> ()
        n172 = local write "Shift Beac"(w404) -> ()
        n173 = Unbundle By Name(w401) -> ("Config.FP_User.3.Cal_"=w386:T11, "Config.FP_User.3.Beac"=w385:T11)
        n174 = local write "SimulateFPGA"(FALSE ("SimulateFPGA")) -> ()
        n175 = local write "84GHz_ctrl"(w400) -> ()
        n176 = local write "72GHz_ctrl"(w400) -> ()
        n177 = Negate(x=w386) -> (-x=w382:T11)
        n178 = local write "Shift Cal 3"(w382) -> ()
        n179 = local write "Shift Beac 3"(w385) -> ()
      }
      frame "Spvsr_RfrshPnl" {
        # "The User level can be used here to configure controls/indicators depending on user privileges."
        # "Use this case to handle all VI panel updates corresponding to program state changes such as enabling/disabling controls based on system states such as HW Mode."
        n180 = call "CheckVariantForClusterUpdate_MainLoop.vi"("ErrorIn"=w416, "VariantIn"=w417, "ClusterIn"=w418) -> ("ErrorOut"=w410:errorcluster, "ClusterOut"=w415:T32)  [unwired: 7 in]
        n181 = Unbundle By Name(w415) -> ("Stat.SysState"=w414:T45, "Admin.Lvl"=w413:T34)
        n182 = case shown="\"Idle\"" w414 {
          tunnel: [T52."Disabled and Grayed Out" ("Disabled") T52."Enabled" ("Disabled") T52."Disabled and Grayed Out" ("Disabled") T52."Disabled and Grayed Out" ("Disabled") T52."Disabled and Grayed Out" ("Disabled") T52."Disabled and Grayed Out" ("Disabled")] -> w411
          tunnel: [T52."Disabled and Grayed Out" ("Disabled") T52."Disabled and Grayed Out" ("Disabled") T52."Disabled and Grayed Out" ("Disabled") T52."Enabled" ("Disabled") T52."Disabled and Grayed Out" ("Disabled") T52."Disabled and Grayed Out" ("Disabled")] -> _
          tunnel: [FALSE FALSE FALSE FALSE TRUE FALSE] -> w409
          frame "Init" {
          }
          frame "Idle" {
          }
          frame "Running" {
          }
          frame "System Fault" {
          }
          frame "System Error" {
          }
          frame "Exit" {
          }
        }
        n183 = case shown="\"Operator\"" w413 {
          frame "Admin", Default {
          }
          frame "Operator" {
          }
        }
        n184 = property on="SysErr" class="Str"(error in=w410, "Visible"=w409) -> (error out=w408:errorcluster)  [unwired: 1 in, 1 out]
        n185 = property on="Stop" class="Bool"(error in=w408, "DisabledEnum"=w411) -> (error out=w412:errorcluster)  [unwired: 1 in, 1 out]
      }
      frame "Spvsr_Cursors" {
        n186 = control-ref of="Beacon"() -> (w452:refnum<vi>)
        n187 = control-ref of="Beacon 2"() -> (w445:refnum<vi>)
        n188 = property class="WFGraph (strict)"(reference=w452, error in=w450) -> (error out=w451:errorcluster, "CrsrList"=w446:T54, "Active Cursor"=w447:u32, "Cursor.Cursor X"=w449:dbl)  [unwired: 1 out]
        n189 = property class="WFGraph (strict)"(reference=w445, error in=w451, "CrsrList"=w446, "Active Cursor"=w447, "Cursor.Cursor X"=w449) -> (error out=w440:errorcluster)  [unwired: 1 out]
        n190 = control-ref of="Beacon 3"() -> (w438:refnum<vi>)
        n191 = control-ref of="Beacon 4"() -> (w437:refnum<vi>)
        n192 = property class="WFGraph (strict)"(reference=w438, error in=w440) -> (error out=w441:errorcluster, "CrsrList"=w444:T54, "Active Cursor"=w443:u32, "Cursor.Cursor X"=w442:dbl)  [unwired: 1 out]
        n193 = property class="WFGraph (strict)"(reference=w437, error in=w441, "CrsrList"=w444, "Active Cursor"=w443, "Cursor.Cursor X"=w442) -> (error out=w439:errorcluster)  [unwired: 1 out]
      }
      frame "Spvsr_Admin" {
        # "This case handles the Admin/Operator menu selection and you can use this to configure your software behavior depending on User Level.  The appropriate place to do this is to read the User Level in the Refresh Panel and set the behavior and appearance of your controls/indicators appropriately."
        n194 = Enqueue Element(queue=w453, element=cluster{"QElmnt":T47, "Data":variant} {"QElmnt"=enum."Spvsr_RfrshPnl", "Data"=variant} ("Cluster"), error in (no error)=w456) -> (error out=w455:errorcluster)  [unwired: 3 out]
        n195 = Unbundle By Name(w463) -> ("Admin.Lvl"=w464:T34, "Admin.Pwd"=w461:string)
        n196 = case shown="\"Operator\", Default" w464 {
          tunnel: w455 -> [w466 w473]
          tunnel: [w466 w469] -> w458
          tunnel: [UserLevelEnum."Operator" ("UserLevel") w470] -> w460
          tunnel: w461 -> [_ w467]
          frame "Admin" {
          }
          frame "Operator", Default {
            n197 = call "AdminLogon.vi"("ErrorIn"=w473, "Password"=w467) -> ("ErrorOut"=w469:errorcluster, "Successful?"=w468:bool)  [unwired: 8 out]
            n198 = Select(t=UserLevelEnum."Admin" ("UserLevel"), s=w468, f=UserLevelEnum."Operator" ("UserLevel")) -> (s? t:f=w470:T34)
          }
        }
        n199 = Current VI's Menubar() -> (w459:refnum<k9>)
        n200 = call "MenuConfiguration.vi"("UserLevel"=w460, "ErrorIn"=w458, "MenuRef"=w459) -> ("ErrorOut"=w457:errorcluster)  [unwired: 8 out]
        n201 = Bundle By Name(cluster=w463, "Admin.Lvl"=w460) -> (w462:T32)
      }
      frame "Spvsr_StrtHWLp" {
        # "If there is a problem with the thresholds file,\ndo not start the AI loop."
        # "Starts the HW Loop and this should only be called once all Main Loop and Software Initialization has occurred to ensure that the HW Loop has the newest data to operate on."
        n202 = Build Array(cluster{"HWMd":T27, "Data":variant} {"HWMd"=enum."HW_Init", "Data"=variant}, cluster{"HWMd":T27, "Data":variant} {"HWMd"=enum."HW_Start", "Data"=variant}, cluster{"HWMd":T27, "Data":variant} {"HWMd"=enum."HW_Run", "Data"=variant}) -> (w483:cluster{"HWMd":T27, "Data":variant}[])
        n203 = call "Init_All_FPGAs.vi"("error in (no error)"=w484, "Array"=w483) -> ("error out"=w478:errorcluster)  [unwired: 9 in]
        n204 = call "PushToErrorHandler.vi"("ErrorIn"=w478, "ErrorLocation"="InitFPGAs") -> ("ErrorOut"=w475:errorcluster)  [unwired: 5 in]
        n205 = Unbundle By Name(w481) -> ("Alarm"=w476:T18, "Config.FP_User.Inclin"=w479:T8)
        n206 = Bundle(cluster=cluster{"Alarm":T18, "Inclin":T8} {"Alarm"={"TC13"={"Enbl"=FALSE, "ErrsAndWarns"={0.0, 0.0, 0.0, 0.0}}, "AI1"={"Enbl"=FALSE, "ErrsAndWarns"={0.0, 0.0, 0.0, 0.0}}, "AI2"={"Enbl"=FALSE, "ErrsAndWarns"={0.0, 0.0, 0.0, 0.0}}, "AI3"={"Enbl"=FALSE, "ErrsAndWarns"={0.0, 0.0, 0.0, 0.0}}, "AI4"={"Enbl"=FALSE, "ErrsAndWarns"={0.0, 0.0, 0.0, 0.0}}, "AI5"={"Enbl"=FALSE, "ErrsAndWarns"={0.0, 0.0, 0.0, 0.0}}, "AI6"={"Enbl"=FALSE, "ErrsAndWarns"={0.0, 0.0, 0.0, 0.0}}, "AI18"={"Enbl"=FALSE, "ErrsAndWarns"={0.0, 0.0, 0.0, 0.0}}, "AI19"={"Enbl"=FALSE, "ErrsAndWarns"={0.0, 0.0, 0.0, 0.0}}, "TE1"={"Enbl"=FALSE, "ErrsAndWarns"={0.0, 0.0, 0.0, 0.0}}, "TE2"={"Enbl"=FALSE, "ErrsAndWarns"={0.0, 0.0, 0.0, 0.0}}, "TE3"={"Enbl"=FALSE, "ErrsAndWarns"={0.0, 0.0, 0.0, 0.0}}, "ADAM1"={"Enbl"=FALSE, "ErrsAndWarns"={0.0, 0.0, 0.0, 0.0}}, "ADAM2"={"Enbl"=FALSE, "ErrsAndWarns"={0.0, 0.0, 0.0, 0.0}}, "ADAM3"={"Enbl"=FALSE, "ErrsAndWarns"={0.0, 0.0, 0.0, 0.0}}, "ADAM4"={"Enbl"=FALSE, "ErrsAndWarns"={0.0, 0.0, 0.0, 0.0}}, "72CoBeacFreq"={"Enbl"=FALSE, "ErrsAndWarns"={0.0, 0.0, 0.0, 0.0}}, "72CoCalFreq"={"Enbl"=FALSE, "ErrsAndWarns"={0.0, 0.0, 0.0, 0.0}}, "84CoBeacFreq"={"Enbl"=FALSE, "ErrsAndWarns"={0.0, 0.0, 0.0, 0.0}}, "84CoCalFreq"={"Enbl"=FALSE, "ErrsAndWarns"={0.0, 0.0, 0.0, 0.0}}, "72Co_CalTonePwr"={"Enbl"=FALSE, "ErrsAndWarns"={0.0, 0.0, 0.0, 0.0}}, "72X_CalTonePwr"={"Enbl"=FALSE, "ErrsAndWarns"={0.0, 0.0, 0.0, 0.0}}, "84Co_CalTonePwr"={"Enbl"=FALSE, "ErrsAndWarns"={0.0, 0.0, 0.0, 0.0}}, "84X_CalTonePwr"={"Enbl"=FALSE, "ErrsAndWarns"={0.0, 0.0, 0.0, 0.0}}}, "Inclin"={"Vmin"=0.0, "Vmax"=0.0, "Angle_min"=0.0, "Angle_max"=0.0, "Offset"=0.0, "Pos_Neg"=FALSE}}, "Alarm"=w476, "Inclin"=w479) -> (w480:cluster{"Alarm":T18, "Inclin":T8})
        n207 = case shown="No Error" w475 {
          tunnel: [w489 errorcluster {"status"=FALSE, "code"=0, "source"=""} ("error out")] -> w482
          tunnel: w480 -> [w488 _]
          frame No Error {
            n208 = To Variant(anything=w488) -> (Variant=w491:variant)
            n209 = Bundle By Name(cluster=cluster{"Enum":T53, "Var":variant} {"Enum"=enum."AI_Init", "Var"=variant}, "Var"=w491) -> (w492:cluster{"Enum":T53, "Var":variant})
            n210 = Build Array("AI" ("name (unnamed)"), "TC" ("name (unnamed)")) -> (w490:string[])
            n211 = for {
              tunnel: w492 -> [w498]
              tunnel: w490 -> [w497] mode=indexing
              shift-right: [w496] -> w489
              shift-left: _ -> [w499]
              n212 = Obtain Queue(max queue size (-1, unlimited)=100, name (unnamed)=w497, element data type=w498, error in (no error)=w499) -> (queue out=w504:refnum<queue>, error out=w502:errorcluster)  [unwired: 1 in, 1 out]
              n213 = Enqueue Element(queue=w504, element=w498, error in (no error)=w502) -> (queue out=w500:refnum<queue>, error out=w501:errorcluster)  [unwired: 1 in, 1 out]
              n214 = Release Queue(queue=w500, error in (no error)=w501) -> (error out=w496:errorcluster)  [unwired: 1 in, 2 out]
            }
          }
          frame Error {
          }
        }
      }
      frame "Spvsr_Stop" {
        # "The Stop case would stop the execution of a currently running test.  The System State is updated and Refresh Panel is called so that the front panel controls can be configured for this state."
        n215 = Enqueue Element(queue=w507, element=cluster{"QElmnt":T47, "Data":variant} {"QElmnt"=enum."Spvsr_RfrshPnl", "Data"=variant} ("Cluster"), error in (no error)=w509) -> (error out=w506:errorcluster)  [unwired: 3 out]
        n216 = Bundle By Name(cluster=w512, "Stat.SysState"=SystemStateEnum."Idle") -> (w511:T32)
      }
      frame "Spvsr_NewData" {
        n217 = Variant To Data(error in=w516, type=T35 {"Arm"=FALSE, "Number"=0.0, "String"=""} ("RTConfig"), Variant=w514) -> (data=w519:T35, error out=w515:errorcluster)
        n218 = Unbundle By Name(w513) -> ("RTConfig"=w518:T35)
        n219 = Equal?(x=w518, y=w519) -> ()  [unwired: 1 out]
      }
      frame "Spvsr_ScaleGraphs" {
        # "no longer allowing user-defined Digital outputs. Digital lines are now controlled programmatically based on error status.\nAO lines are user controlled.\n\nLuke 12-15-2017"
      }
      frame "Spvsr_Error" {
        # "The Error Handler case can be called from anywhere in the software and is called using the PushToErrorHandler.vi.  This allows for the software to handle errors in one spot in the software while allowing the Main Loop to push a new state to the HW and other loops.  Note that for the user defined error code 5000, conditions (HW Disabled) are set, an event is sent down to instantly reconfigure the system and THEN the message dialog box can be popped up for the user.  In some cases, you may not want to popup a dialog box (as shown below for 5000), but merely clear an error and reset or pause hardware. \n\nIt is an impossible task to define exactly how all software should behave with respect to handling error, but the most important thing is that as a developer, you must consider all possible sources of error and to ensure that your software responds appropriately.  The PushToErrorHandler.vi should be used frequently to ensure that you trap all errors as if there is a potential for an error to occur, you should consider how your software will behave when that error occurs and how you need/want to present this error to the user."
